vi "GetAvailableData.vi"(6 "Delay between send and receive [ms]":i32=100, 8 "error in (no error)":errorcluster, 10 "Channels to be requested":T1[](array[typedef]), 11 "SCD in":refnum<class "SCD.lvclass">) -> (0 "error out":errorcluster, 2 "data":T2(array[cluster]), 3 "SCD out":refnum<class "SCD.lvclass">)   [LabVIEW 2020, in "horiba.lvlib" / "SCD.lvclass"]
doc: "Check whether the acquired data is available."
uses:
  SCD.lvclass
  dataChannels.ctl
  scdData.ctl
  b6349250-cb33-415b-847a-a7f5d99734f6.vi
  a3575502-22b1-481e-8bb0-96f3cfd6d110.vi
  <vilib>/JDP Science/JSONtext/Variant to JSON Text.vi
  <vilib>/JDP Science/JSONtext/Set Item.vi
  <vilib>/JDP Science/JSONtext/JSON text to Variant.vi
  <vilib>/JDP Science/JSONtext/LVClass Serializer/JSONtext LVClass Serializer.lvclass
  GenericDevice/GenericDevice.lvclass
panel:
  # "Connector Pane"
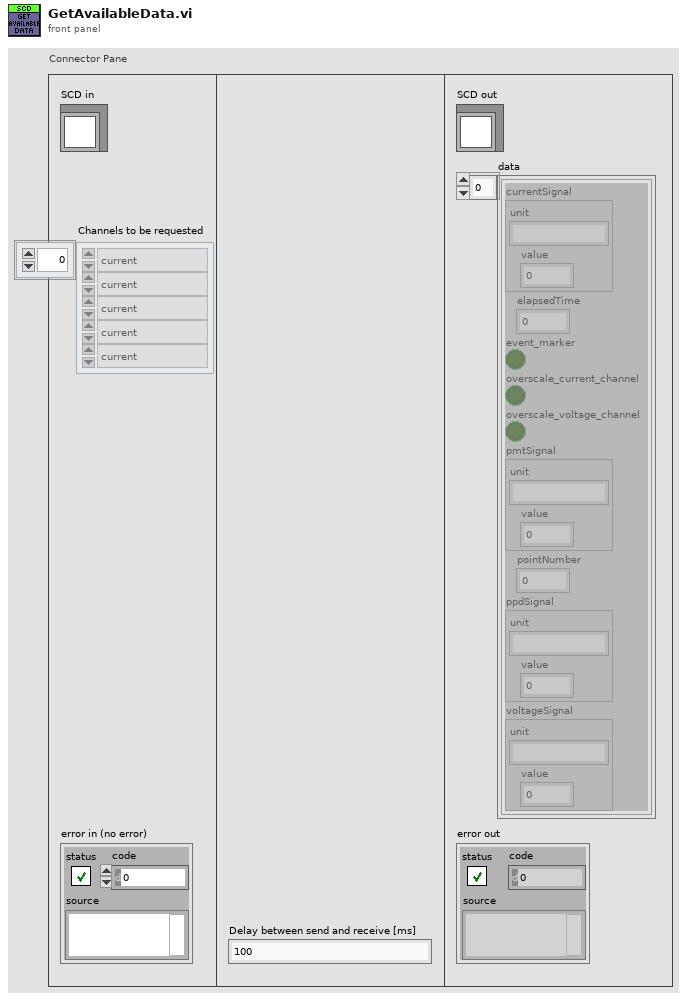
[diagram p1: front panel]
types:
  T1 = typedef "horiba.lvlib/SCD.lvclass/dataChannels.ctl" = enum16{"current", "voltage", "ppd", "photon"}
  T2 = cluster{"currentSignal":cluster{"unit":string, "value":dbl}, "elapsedTime":dbl, "event_marker":bool, "overscale_current_channel":bool, "overscale_voltage_channel":bool, "pmtSignal":cluster{"unit":string, "value":dbl}, "pointNumber":dbl, "ppdSignal":cluster{"unit":string, "value":dbl}, "voltageSignal":cluster{"unit":string, "value":dbl}}[]
  T3 = typedef "horiba.lvlib/SCD.lvclass/scdData.ctl" = cluster{"data":cluster{"currentSignal":cluster{"unit":string, "value":dbl}, "elapsedTime":dbl, "event_marker":bool, "overscale_current_channel":bool, "overscale_voltage_channel":bool, "pmtSignal":cluster{"unit":string, "value":dbl}, "pointNumber":dbl, "ppdSignal":cluster{"unit":string, "value":dbl}, "voltageSignal":cluster{"unit":string, "value":dbl}}[]}
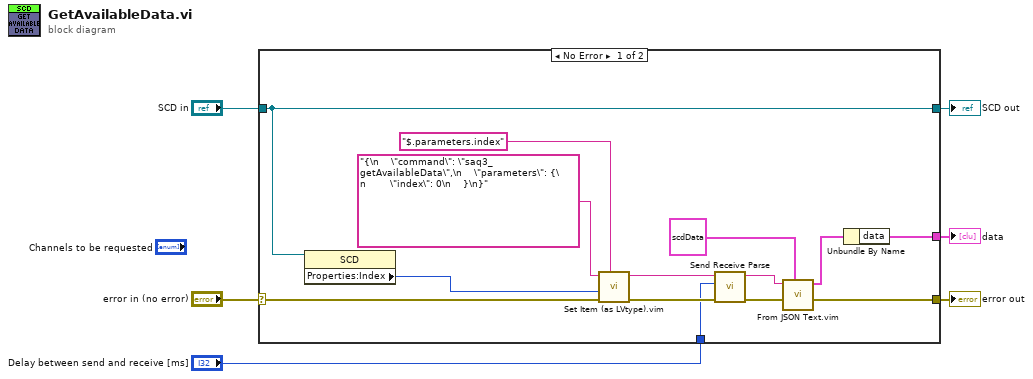
[diagram p0: block diagram]
diagram:
  n1 = case shown="No Error" "error in (no error)" {
    selector: "error in (no error)" -> [w16 w22]
    tunnel: [w15 w22] -> w2
    tunnel: [w18 w21] -> w4
    tunnel: "SCD in" -> [w18 w21]
    tunnel: [w10 _] -> w1
    tunnel: "Delay between send and receive [ms]" -> [w9 _]
    frame No Error {
      n2 = property class="SCD"(reference=w18) -> ("Properties:Index"=w17:i32)  [unwired: 1 in, 2 out]
      n3 = call "Set Item (as LVtype).vim"("$Path or Item Name"="$.parameters.index", "error in (no error)"=w16, "Anything"=w17, "JSON"="{\n    \"command\": \"saq3_getAvailableData\",\n    \"parameters\": {\n        \"index\": 0\n    }\n}") -> ("error out"=w13:errorcluster, "<JSON>"=w8:string)  [unwired: 4 in, 1 out]
      n4 = call "Send Receive Parse.vi"("error in"=w13, "Delay between send and receive [ms]"=w9, "<JSON>"=w8) -> ("error out"=w12:errorcluster, "results-JSON string"=w14:string)  [unwired: 6 in, 1 out]
      n5 = call "From JSON Text.vim"("Data Type and Default Value"=T3 {"data"=[{"currentSignal"={"unit"="", "value"=0.0}, "elapsedTime"=0.0, "event_marker"=FALSE, "overscale_current_channel"=FALSE, "overscale_voltage_channel"=FALSE, "pmtSignal"={"unit"="", "value"=0.0}, "pointNumber"=0.0, "ppdSignal"={"unit"="0", "value"=0.0}, "voltageSignal"={"unit"="", "value"=0.0}}]} ("scdData"), "error in (no error)"=w12, "JSON"=w14) -> ("error out"=w15:errorcluster, "Data out"=w11:T3)  [unwired: 7 in]
      n6 = Unbundle By Name(w11) -> ("data"=w10:T2)
    }
    frame Error {
    }
  }
  "error out" <- w2
  "SCD out" <- w4
  "data" <- w1
